vi "AddProduct.vi"(7 "error in (no error)":errorcluster) -> (0 "error out":errorcluster, 1 "Cancelled?":bool, 3 "New Product":T1)   [LabVIEW 2020]
doc: "VI adds new product. Cancelled? indicator equals true if operation was cancelled"
uses:
  #typedef_Product.ctl
panel:
  in  "Cancel":bool
  in  "OK":bool
  in  "Product":T1
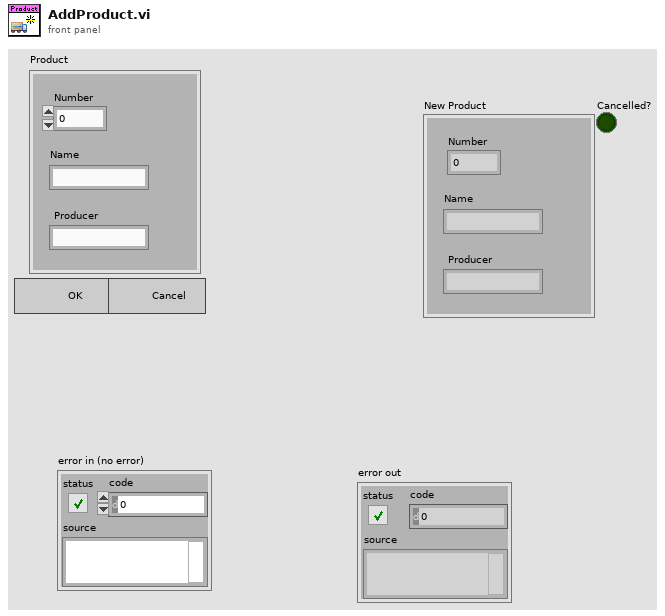
[diagram p1: front panel]
types:
  T1 = typedef "#typedef_Product.ctl" = cluster{"Number":i32, "Name":string, "Producer":string}
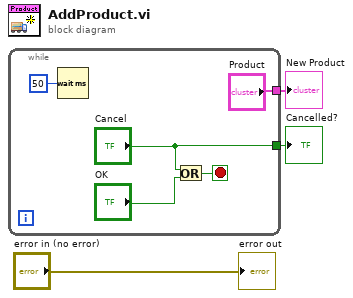
[diagram p0: block diagram]
diagram:
  n1 = while {
    tunnel: ["Product"] -> w3
    tunnel: ["Cancel"] -> w2
    stop <- w7 stop-if-true
    n2 = Wait (ms)(milliseconds to wait=u32 50 ("millisecond timer value")) -> ()  [unwired: 1 out]
    n3 = Or(x="Cancel", y="OK") -> (x .or. y?=w7:bool)
  }
  "New Product" <- w3
  "Cancelled?" <- w2
  "error out" <- "error in (no error)"
